vi "Analytical Inverse Kinematics (6R Type 3).vi"(8 "error in (no error)":errorcluster, 10 "end effector transform":T1, 11 "6R type 3 serial arm in":refnum<class "NI_Robotics_6R Type 3 Serial Arm Class.lvclass">) -> (0 "error out":errorcluster, 1 "number of valid solutions":i32, 2 "joint positions":T1, 3 "6R type 3 serial arm out":refnum<class "NI_Robotics_6R Type 3 Serial Arm Class.lvclass">)   [LabVIEW 2017, in "NI_Robotics_6R Type 3 Serial Arm Class.lvclass"]
doc: "Returns the joint angles of a 6R, 5R, or SCARA arm given the posture of the end effector relative to the arm base. Wire data to the <B>X</B><B>_serial arm in</B> input, where <B>X</B> is the arm type, to determine the polymorphic instance to use or manually select the instance."
uses:
  <vilib>/robotics/Kinematics/Analytical/6R/Type 3/NI_Robotics_6R Type 3 Serial Arm Class.lvclass
  c:/Program Files (x86)/National Instruments/LabVIEW 2017/vi.lib/robotics/Kinematics/Robot/NI_Robotics_Serial Robot Arm.lvclass
  c:/Program Files (x86)/National Instruments/LabVIEW 2017/vi.lib/robotics/Kinematics/Analytical/Generic/NI_Robotics_Analytical Serial Arm Class.lvclass
  <vilib>/Analysis/Matrix/Datatypes/RealMatrix.ctl
  <vilib>/Analysis/baseanly.llb/Real A x B.vi
  <vilib>/Analysis/baseanly.llb/Real Inverse Matrix.vi
  <vilib>/robotics/Kinematics/Robot/NI_Robotics_Serial Robot Arm.lvclass
  <vilib>/Analysis/NI_AALBase.lvlib
  <vilib>/robotics/Kinematics/NI_Kinematics.lvlib
  <vilib>/robotics/Kinematics/Analytical/Generic/NI_Robotics_Analytical Serial Arm Class.lvclass
  <vilib>/Analysis/Matrix/NI_Matrix.lvlib
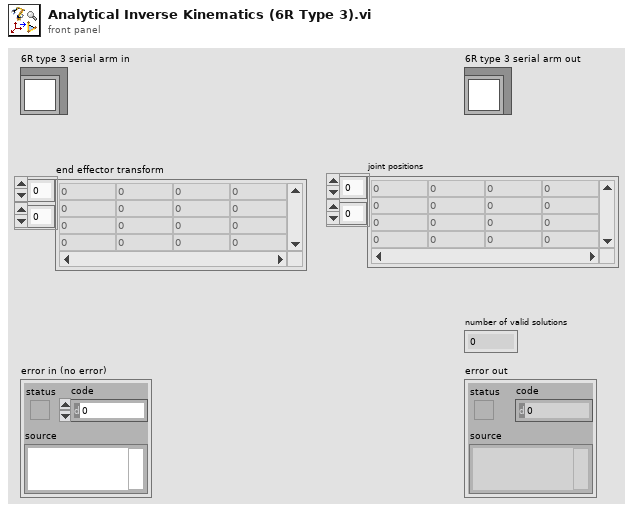
[diagram p1: front panel]
types:
  T1 = typedef "NI_Matrix.lvlib/RealMatrix.ctl" = dbl[][]
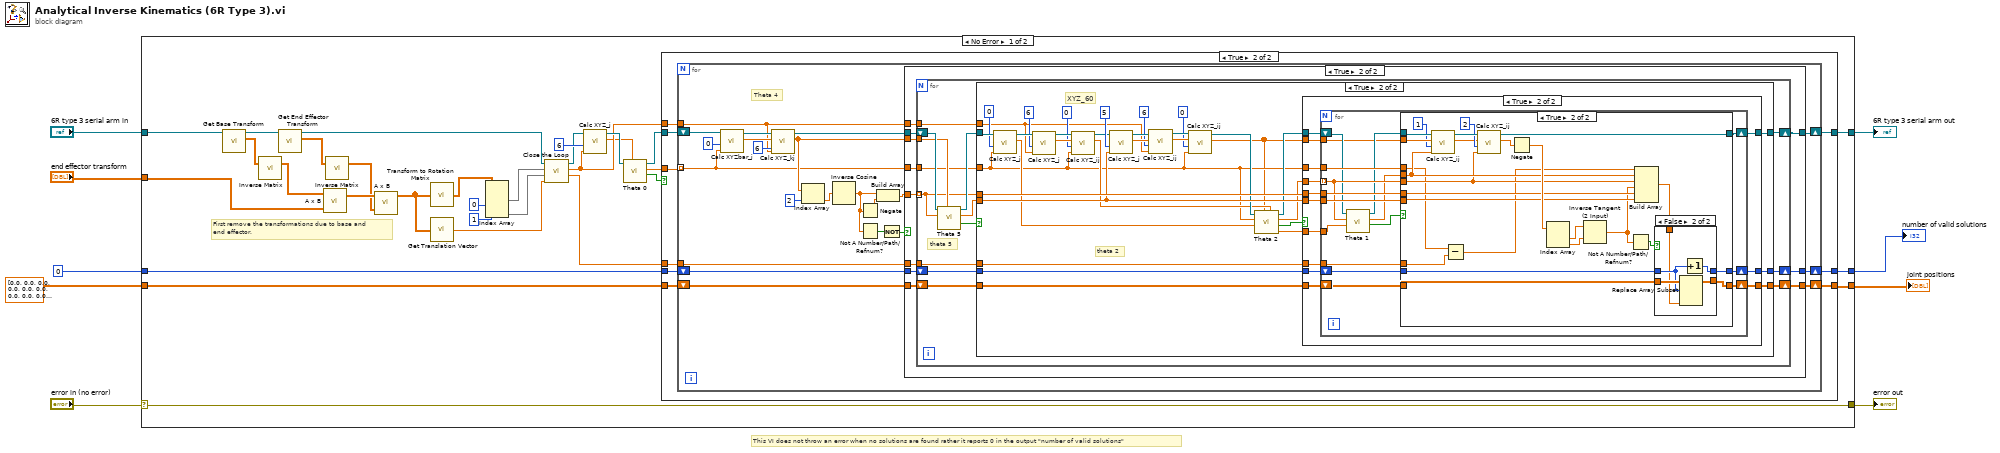
[diagram p0: block diagram]
diagram:
  # "This VI does not throw an error when no solutions are found rather it reports 0 in the output \"number of valid solutions\""
  n1 = case shown="No Error" "error in (no error)" {
    selector: "error in (no error)" -> [w40 w207]
    tunnel: [w40 w207] -> w8
    tunnel: [w24 w206] -> w6
    tunnel: "6R type 3 serial arm in" -> [w21 w206]
    tunnel: "end effector transform" -> [w25 _]
    tunnel: dbl[][] [[0.0, 0.0, 0.0, 0.0, 0.0, 0.0], [0.0, 0.0, 0.0, 0.0, 0.0, 0.0], [0.0, 0.0, 0.0, 0.0, 0.0, 0.0], [0.0, 0.0, 0.0, 0.0, 0.0, 0.0], [0.0, 0.0, 0.0, 0.0, 0.0, 0.0], [0.0, 0.0, 0.0, 0.0, 0.0, 0.0], [0.0, 0.0, 0.0, 0.0, 0.0, 0.0], [0.0, 0.0, 0.0, 0.0, 0.0, 0.0]] ("Solutions") -> [w22 _]
    tunnel: 0 -> [w23 _]
    tunnel: [w13 _] -> w2
    tunnel: [w12 _] -> w1
    frame No Error {
      # "First remove the transformations due to base and\nend effector."
      n2 = call <vilib>:"Get Base Transform.vi"("serial arm in"=w21) -> ("base transform"=w37:T1, "serial arm out"=w39:refnum<class "NI_Robotics_6R Type 3 Serial Arm Class.lvclass">)  [unwired: 8 in, 1 out]
      n3 = call-poly <vilib>:"Inverse Matrix.vi"("Input Matrix"=w37) -> ("Inverse Matrix"=w36:T1)  [unwired: 1 in, 1 out]
      n4 = call <vilib>:"Get End Effector Transform.vi"("serial arm in"=w39) -> ("end effector transform"=w38:T1, "serial arm out"=w32:refnum<class "NI_Robotics_6R Type 3 Serial Arm Class.lvclass">)  [unwired: 8 in, 1 out]
      n5 = call-poly <vilib>:"A x B.vi"("B"=w25, "A"=w36) -> ("A x B"=w35:T1)  [unwired: 1 out]
      n6 = call-poly <vilib>:"Inverse Matrix.vi"("Input Matrix"=w38) -> ("Inverse Matrix"=w34:T1)  [unwired: 1 in, 1 out]
      n7 = call-poly <vilib>:"A x B.vi"("B"=w34, "A"=w35) -> ("A x B"=w33:T1)  [unwired: 1 out]
      n8 = call <vilib>:"Transform to Rotation Matrix.vi"("transform"=w33) -> ("rotation matrix"=w28:T1)
      n9 = call <vilib>:"Get Translation Vector.vi"("transform"=w33) -> ("translation vector"=w31:dbl[])
      n10 = Index Array(array=w28, index (col) #1=0 ("disabled index (col)"), index (col) #2=1 ("index (col)")) -> (element #1=w26:dbl[], element #2=w27:dbl[])  [unwired: 2 in]
      n11 = call <vilib>:"Close the Loop.vi"("P_toolf"=w31, "S_n-1f"=w27, "a_(n-1)nf"=w26, "Analytical Serial Arm Class in"=w32) -> ("gamma_0"=w19:dbl, "theta_n"=w16:dbl, "Analytical Serial Arm Class out"=w18:refnum<class "NI_Robotics_6R Type 3 Serial Arm Class.lvclass">)  [unwired: 5 in]
      n12 = call <vilib>:"Calc XYZ_j.vi"("theta_j"=w16, "j"=6, "Analytical Serial Arm Class in"=w18) -> ("XYZ_j"=w15:dbl[], "Analytical Serial Arm Class out"=w17:refnum<class "NI_Robotics_6R Type 3 Serial Arm Class.lvclass">)  [unwired: 7 in]
      n13 = call <vilib>:"Theta 0.vi"("XYZ_6"=w15, "6R Type 3 Serial Arm Class.lvclass"=w17) -> ("valid?"=w10:bool, "theta_0 array"=w14:dbl[], "6R Type 3 Serial Arm Class.lvclass out"=w11:refnum<class "NI_Robotics_6R Type 3 Serial Arm Class.lvclass">)  [unwired: 7 in]
      n14 = case shown="True" w10 {
        tunnel: [w43 w52] -> w24
        tunnel: w23 -> [w42 w51]
        tunnel: w22 -> [w41 w50]
        tunnel: w19 -> [_ w49]
        tunnel: w16 -> [_ w48]
        tunnel: w14 -> [_ w47]
        tunnel: [w42 w46] -> w12
        tunnel: [w41 w45] -> w13
        tunnel: w11 -> [w43 w44]
        frame False {
        }
        frame True {
          n15 = for {
            tunnel: w47 -> [w54] mode=indexing
            tunnel: w48 -> [w53]
            shift-right: [w59] -> w52
            shift-left: w44 -> [w69]
            tunnel: w49 -> [w74]
            shift-right: [w70] -> w45
            shift-left: w50 -> [w72]
            shift-right: [w71] -> w46
            shift-left: w51 -> [w73]
            # "Theta 4"
            n16 = call <vilib>:"Calc XYZbar_j.vi"("theta_j"=w54, "j"=0, "Analytical Serial Arm Class in"=w69) -> ("XYZbar_j"=w67:dbl[], "Analytical Serial Arm Class out"=w68:refnum<class "NI_Robotics_6R Type 3 Serial Arm Class.lvclass">)  [unwired: 7 in]
            n17 = call <vilib>:"Calc XYZ_kj.vi"("theta_j"=w53, "j"=6, "XYZbar_k"=w67, "Analytical Serial Arm Class in"=w68) -> ("XYZ_ij"=w58:dbl[], "Analytical Serial Arm Class out"=w60:refnum<class "NI_Robotics_6R Type 3 Serial Arm Class.lvclass">)  [unwired: 5 in, 1 out]
            n18 = Index Array(array=w58, index=2) -> (element=w64:dbl)
            n19 = Inverse Cosine(1:w64) -> (0:w57:dbl)
            n20 = Negate(x=w57) -> (-x=w61:dbl)
            n21 = Not A Number/Path/Refnum?(number/path/refnum=w57) -> (NaN/Path/Refnum?=w56:bool)
            n22 = Build Array(w57, w61) -> (w62:dbl[])
            n23 = Not(x=w56) -> (.not. x?=w55:bool)
            n24 = case shown="True" w55 {
              tunnel: w54 -> [_ w86]
              tunnel: w60 -> [w77 w88]
              tunnel: [w77 w87] -> w59
              tunnel: w62 -> [_ w78]
              tunnel: w58 -> [_ w85]
              tunnel: w74 -> [_ w84]
              tunnel: w53 -> [_ w83]
              tunnel: w73 -> [w76 w82]
              tunnel: w72 -> [w75 w81]
              tunnel: [w76 w80] -> w71
              tunnel: [w75 w79] -> w70
              frame False {
              }
              frame True {
                n25 = for {
                  shift-right: [w89] -> w87
                  shift-left: w88 -> [w96]
                  tunnel: w78 -> [w93] mode=indexing
                  tunnel: w86 -> [w90]
                  tunnel: w85 -> [w94]
                  tunnel: w84 -> [w102]
                  tunnel: w83 -> [w101]
                  shift-right: [w97] -> w79
                  shift-left: w81 -> [w99]
                  shift-right: [w98] -> w80
                  shift-left: w82 -> [w100]
                  # "theta 5"
                  n26 = call <vilib>:"Theta 5.vi"("XYZ_6"=w94, "theta_4"=w93, "6R Type 3 Serial Arm Class in"=w96) -> ("valid?"=w92:bool, "theta_5"=w91:dbl, "6R Type 3 Serial Arm Class out"=w95:refnum<class "NI_Robotics_6R Type 3 Serial Arm Class.lvclass">)  [unwired: 6 in]
                  n27 = case shown="True" w92 {
                    tunnel: [w103 w138] -> w89
                    tunnel: w102 -> [_ w136]
                    tunnel: w101 -> [_ w116]
                    tunnel: w100 -> [w105 w135]
                    tunnel: w99 -> [w104 w137]
                    tunnel: [w105 w134] -> w98
                    tunnel: [w104 w133] -> w97
                    tunnel: w95 -> [w103 w131]
                    tunnel: w93 -> [_ w132]
                    tunnel: w91 -> [_ w126]
                    tunnel: w90 -> [_ w108]
                    frame False {
                    }
                    frame True {
                      # "XYZ_60"
                      # "theta 2"
                      n28 = call <vilib>:"Calc XYZ_j.vi"("theta_j"=w108, "j"=0, "Analytical Serial Arm Class in"=w131) -> ("XYZ_j"=w113:dbl[], "Analytical Serial Arm Class out"=w129:refnum<class "NI_Robotics_6R Type 3 Serial Arm Class.lvclass">)  [unwired: 7 in]
                      n29 = call <vilib>:"Calc XYZ_j.vi"("theta_j"=w116, "j"=6, "Analytical Serial Arm Class in"=w129) -> ("XYZ_j"=w124:dbl[], "Analytical Serial Arm Class out"=w125:refnum<class "NI_Robotics_6R Type 3 Serial Arm Class.lvclass">)  [unwired: 7 in]
                      n30 = call <vilib>:"Calc XYZ_ij.vi"("theta_j"=w108, "j"=0, "XYZ_i"=w124, "Analytical Serial Arm Class in"=w125) -> ("XYZ_ij"=w112:dbl[], "Analytical Serial Arm Class out"=w122:refnum<class "NI_Robotics_6R Type 3 Serial Arm Class.lvclass">)  [unwired: 5 in, 1 out]
                      n31 = call <vilib>:"Calc XYZ_j.vi"("theta_j"=w126, "j"=5, "Analytical Serial Arm Class in"=w122) -> ("XYZ_j"=w121:dbl[], "Analytical Serial Arm Class out"=w120:refnum<class "NI_Robotics_6R Type 3 Serial Arm Class.lvclass">)  [unwired: 7 in]
                      n32 = call <vilib>:"Calc XYZ_ij.vi"("theta_j"=w116, "j"=6, "XYZ_i"=w121, "Analytical Serial Arm Class in"=w120) -> ("XYZ_ij"=w118:dbl[], "Analytical Serial Arm Class out"=w117:refnum<class "NI_Robotics_6R Type 3 Serial Arm Class.lvclass">)  [unwired: 5 in, 1 out]
                      n33 = call <vilib>:"Calc XYZ_ij.vi"("theta_j"=w108, "j"=0, "XYZ_i"=w118, "Analytical Serial Arm Class in"=w117) -> ("XYZ_ij"=w106:dbl[], "Analytical Serial Arm Class out"=w114:refnum<class "NI_Robotics_6R Type 3 Serial Arm Class.lvclass">)  [unwired: 5 in, 1 out]
                      n34 = call <vilib>:"Theta 2.vi"("XYZ_60"=w112, "XYZ_560"=w106, "XYZ_0"=w113, "theta_0"=w108, "6R Type 3 Serial Arm Class in"=w114) -> ("AB"=w107:dbl[], "valid?"=w111:bool, "theta_0 array"=w109:dbl[], "6R Type 3 Serial Arm Class out"=w110:refnum<class "NI_Robotics_6R Type 3 Serial Arm Class.lvclass">)  [unwired: 3 in]
                      n35 = case shown="True" w111 {
                        tunnel: w110 -> [w141 w154]
                        tunnel: [w141 w153] -> w138
                        tunnel: w108 -> [_ w151]
                        tunnel: w109 -> [_ w150]
                        tunnel: w132 -> [_ w152]
                        tunnel: w137 -> [w139 w149]
                        tunnel: w136 -> [_ w148]
                        tunnel: w135 -> [w140 w147]
                        tunnel: [w140 w146] -> w134
                        tunnel: [w139 w145] -> w133
                        tunnel: w126 -> [_ w144]
                        tunnel: w107 -> [_ w143]
                        tunnel: w106 -> [_ w142]
                        frame False {
                        }
                        frame True {
                          n36 = for {
                            shift-right: [w155] -> w153
                            shift-left: w154 -> [w160]
                            tunnel: w152 -> [w170]
                            tunnel: w151 -> [w164]
                            tunnel: w150 -> [w162] mode=indexing
                            tunnel: w148 -> [w168]
                            shift-right: [w166] -> w145
                            shift-left: w149 -> [w169]
                            shift-right: [w165] -> w146
                            shift-left: w147 -> [w167]
                            tunnel: w144 -> [w163]
                            tunnel: w143 -> [w161]
                            tunnel: w142 -> [w156]
                            n37 = call <vilib>:"Theta 1.vi"("AB"=w161, "theta_2"=w162, "6R Type 3 Serial Arm Class in"=w160) -> ("valid?"=w157:bool, "theta_1"=w158:dbl, "6R Type 3 Serial Arm Class out"=w159:refnum<class "NI_Robotics_6R Type 3 Serial Arm Class.lvclass">)  [unwired: 6 in]
                            n38 = case shown="True" w157 {
                              tunnel: w159 -> [w173 w189]
                              tunnel: [w173 w182] -> w155
                              tunnel: w170 -> [_ w179]
                              tunnel: w169 -> [w171 w192]
                              tunnel: w168 -> [_ w196]
                              tunnel: w167 -> [w172 w193]
                              tunnel: [w171 w191] -> w166
                              tunnel: [w172 w190] -> w165
                              tunnel: w162 -> [_ w176]
                              tunnel: w164 -> [_ w175]
                              tunnel: w163 -> [_ w180]
                              tunnel: w158 -> [_ w177]
                              tunnel: w156 -> [_ w188]
                              frame False {
                              }
                              frame True {
                                n39 = call <vilib>:"Calc XYZ_ij.vi"("theta_j"=w177, "j"=1, "XYZ_i"=w188, "Analytical Serial Arm Class in"=w189) -> ("XYZ_ij"=w184:dbl[], "Analytical Serial Arm Class out"=w186:refnum<class "NI_Robotics_6R Type 3 Serial Arm Class.lvclass">)  [unwired: 5 in, 1 out]
                                n40 = Subtract(x=w175, y=w196) -> (x-y=w174:dbl)
                                n41 = call <vilib>:"Calc XYZ_ij.vi"("theta_j"=w176, "j"=2, "XYZ_i"=w184, "Analytical Serial Arm Class in"=w186) -> ("XYZ_ij"=w183:dbl[], "Analytical Serial Arm Class out"=w182:refnum<class "NI_Robotics_6R Type 3 Serial Arm Class.lvclass">)  [unwired: 5 in, 1 out]
                                n42 = Negate(x=w183) -> (-x=w181:dbl[])
                                n43 = Index Array(array=w181) -> (element #1=w198:dbl, element #2=w197:dbl)  [unwired: 2 in]
                                n44 = Inverse Tangent (2 Input)(1:w197, 2:w198) -> (0:w178:dbl)
                                n45 = Not A Number/Path/Refnum?(number/path/refnum=w178) -> (NaN/Path/Refnum?=w195:bool)
                                n46 = Build Array(w174, w177, w176, w178, w179, w180) -> (w194:dbl[])
                                n47 = case shown="False" w195 {
                                tunnel: w192 -> [w199 w205]
                                tunnel: [w199 w204] -> w191
                                tunnel: w193 -> [w200 w203]
                                tunnel: [w200 w202] -> w190
                                tunnel: w194 -> [_ w201]
                                frame True {
                                }
                                frame False {
                                n48 = Replace Array Subset(array=w205, new element=w201, index (row)=w203) -> (w204:dbl[][])  [unwired: 1 in]
                                n49 = Increment(x=w203) -> (x+1=w202:i32)
                                }
                                }
                              }
                            }
                          }
                        }
                      }
                    }
                  }
                }
              }
            }
          }
        }
      }
    }
    frame Error {
    }
  }
  "error out" <- w8
  "6R type 3 serial arm out" <- w6
  "joint positions" <- w2
  "number of valid solutions" <- w1
